vi "Numeric Controls.vi"() -> ()   [LabVIEW 2016]
uses:
  QD Code/Templates/NC Templates/sgl.ctl
  QD Code/Templates/NC Templates/dbl.ctl
  QD Code/Templates/NC Templates/ext.ctl
  QD Code/Templates/NC Templates/u8.ctl
  QD Code/Templates/NC Templates/u16.ctl
  QD Code/Templates/NC Templates/u32.ctl
  QD Code/Templates/NC Templates/u64.ctl
  QD Code/Templates/NC Templates/i8.ctl
  QD Code/Templates/NC Templates/i16.ctl
  QD Code/Templates/NC Templates/i32.ctl
  QD Code/Templates/NC Templates/i64.ctl
panel:
  in  "I64":T1
  in  "I32":T2
  in  "I16":T3
  in  "I8":T4
  in  "U64":T5
  in  "U32":T6
  in  "U16":T7
  in  "U8":T8
  in  "EXT":T9
  in  "DBL":T10
  in  "SGL":T11
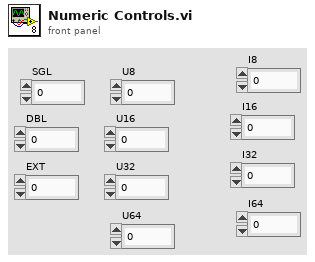
[diagram p1: front panel]
types:
  T1 = typedef "i64.ctl" = i64
  T2 = typedef "i32.ctl" = i32
  T3 = typedef "i16.ctl" = i16
  T4 = typedef "i8.ctl" = i8
  T5 = typedef "u64.ctl" = u64
  T6 = typedef "u32.ctl" = u32
  T7 = typedef "u16.ctl" = u16
  T8 = typedef "u8.ctl" = u8
  T9 = typedef "ext.ctl" = ext
  T10 = typedef "dbl.ctl" = dbl
  T11 = typedef "sgl.ctl" = sgl
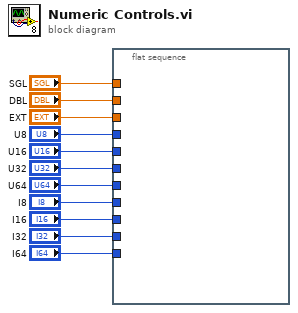
[diagram p0: block diagram]
diagram:
  n1 = flat-sequence {
    tunnel: "I64" -> [_]
    tunnel: "I32" -> [_]
    tunnel: "I16" -> [_]
    tunnel: "I8" -> [_]
    tunnel: "U64" -> [_]
    tunnel: "U32" -> [_]
    tunnel: "U16" -> [_]
    tunnel: "U8" -> [_]
    tunnel: "EXT" -> [_]
    tunnel: "DBL" -> [_]
    tunnel: "SGL" -> [_]
    frame #0 {
    }
  }
